vi "ExSubCloseImageDisplay.vi"(1 "error in (no error)":errorcluster, 2 "Handles In":T1) -> (0 "error out":errorcluster)   [LabVIEW 2010]
panel:
  # "ExSubCloseImageDisplay:\nThis is a subVI which takes a cluster of handles and closes the display, and image only"
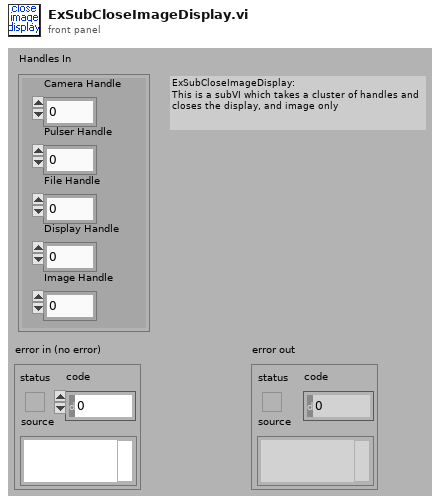
[diagram p1: front panel]
types:
  T1 = cluster{"Camera Handle":u32, "Pulser Handle":u32, "File Handle":u32, "Display Handle":u32, "Image Handle":u32}
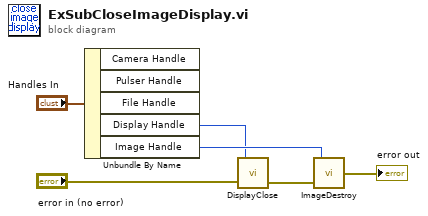
[diagram p0: block diagram]
diagram:
  n1 = Unbundle By Name("Handles In") -> ("Display Handle"=w4:u32, "Image Handle"=w5:u32)  [unwired: 3 out]
  n2 = call <userlib>:"DisplayClose.vi"("error in"="error in (no error)", "Display Handle"=w4) -> ("error out"=w3:errorcluster)
  n3 = call <userlib>:"ImageDestroy.vi"("error in"=w3, "Data handle"=w5) -> ("error out"=→"error out":errorcluster)
